vi "RGB To ARGB.vi"(10 "Depth":i32, 11 "Image Data":u8[](array[numeric])) -> (3 "RGBA":u8[](array[numeric]))   [LabVIEW 2020, in "G-Image.lvlib"]
doc: "Convert the image memory layout from RGB or ARGB to RGBA. Applies to 24-bit and 32-bit images only."
uses:
  G-Image.lvlib
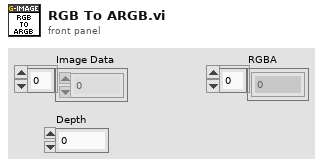
[diagram p1: front panel]
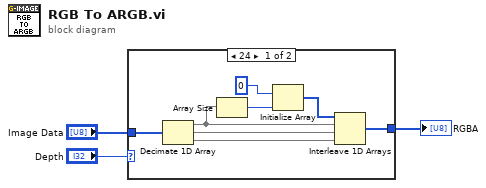
[diagram p0: block diagram]
diagram:
  n1 = case shown="24" "Depth" {
    tunnel: "Image Data" -> [w11 w12]
    tunnel: [w10 w12] -> w1
    frame 24 {
      n2 = Decimate 1D Array(w11) -> (w5:u8[], w9:u8[], w7:u8[])
      n3 = Array Size(array=w5) -> (size(s)=w8:i32)
      n4 = Initialize Array(u8 0, w8) -> (w4:u8[])
      n5 = Interleave 1D Arrays(w4, w5, w9, w7) -> (w10:u8[])
    }
    frame Default {
      # "1, 4, 8, 32"
    }
  }
  "RGBA" <- w1
